vi "GetInstrumentPaths.vi"(8 "Instrument":string, 11 "Build?":bool=TRUE) -> (0 "Path To Raw Folder":path, 1 "Path To Test Folder":path, 2 "Path to csv Folder":path, 3 "Path To Instrument Folder":path, 4 "Path To TRF Folder":path)   [LabVIEW 2022 SP3]
uses:
  Mic/Mic_Global.vi
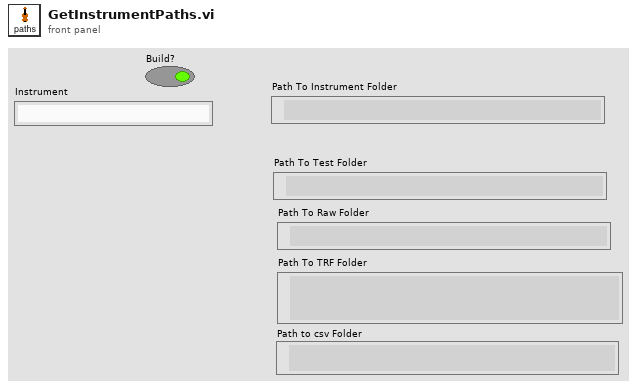
[diagram p1: front panel]
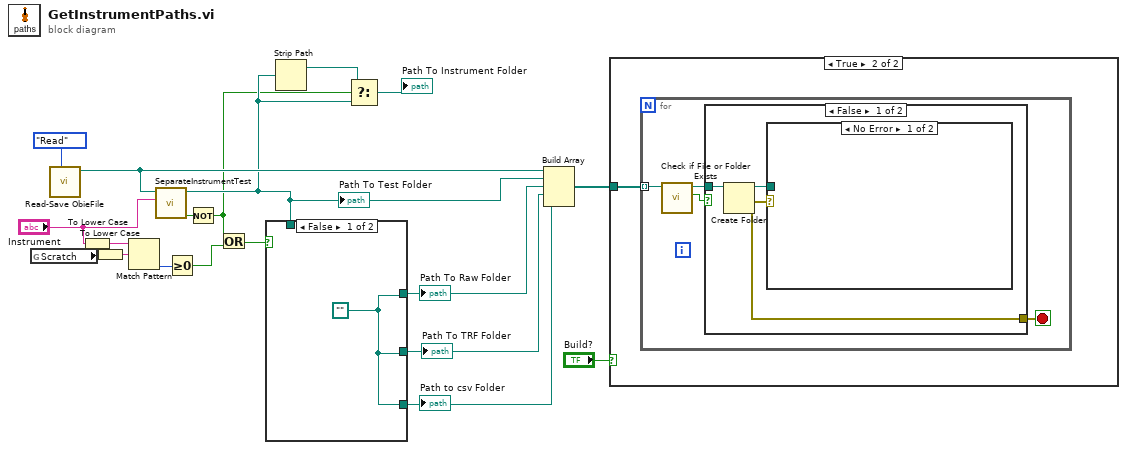
[diagram p0: block diagram]
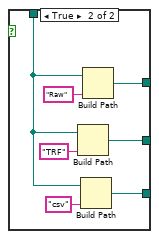
[diagram p5: hidden frame]
diagram:
  n1 = global read "Mic_Global.vi" "Scratch"() -> (w6:string)
  n2 = call "Read-Save ObieFile.vi"("Task"=enum16{"Save", "Read"}."Read") -> ("DataPath Out"=w17:path)  [unwired: 8 in, 2 out]
  n3 = To Lower Case(string="Instrument") -> (all lower case string=w2:string)
  n4 = To Lower Case(string=w6) -> (all lower case string=w1:string)
  n5 = Match Pattern(string=w2, regular expression=w1) -> (offset past match=w4:i32)  [unwired: 1 in, 3 out]
  n6 = call "SeparateInstrumentTest.vi"("Instrument"="Instrument", "path in"=w17) -> ("Single Folder?"=w11:bool, "path out"=w13:path)  [unwired: 5 in, 3 out]
  "Path To Test Folder" <- w13
  n7 = Greater Or Equal To 0?(x=w4) -> (x >= 0?=w3:bool)
  n8 = Not(x=w11) -> (.not. x?=w9:bool)
  n9 = Or(x=w9, y=w3) -> (x .or. y?=w10:bool)
  n10 = case shown="False" w10 {
    tunnel: [w20 w26] -> w16
    tunnel: [w20 w24] -> w15
    tunnel: w13 -> [_ w22]
    tunnel: [w20 w21] -> w8
    frame False {
      w20 = path ""
    }
    frame True {
      n11 = Build Path(base path=w22, name or relative path="TRF") -> (appended path=w24:path)
      n12 = Build Path(base path=w22, name or relative path="csv") -> (appended path=w21:path)
      n13 = Build Path(base path=w22, name or relative path="Raw") -> (appended path=w26:path)
    }
  }
  "Path To Raw Folder" <- w16
  "Path To TRF Folder" <- w15
  "Path to csv Folder" <- w8
  n14 = Strip Path(path=w13) -> (stripped path=w14:path)  [unwired: 1 out]
  n15 = Select(t=w14, s=w9, f=w13) -> (s? t:f=→"Path To Instrument Folder":path)
  n16 = Build Array(w17, w13, w16, w15, w8) -> (w19:path[])
  n17 = case shown="True" "Build?" {
    tunnel: w19 -> [_ w28]
    frame False {
    }
    frame True {
      n18 = for {
        tunnel: w28 -> [w30] mode=indexing
        stop <- w29 stop-if-true
        n19 = call <vilib>:"Check if File or Folder Exists.vi"("path"=w30) -> ("file or folder exists?"=w31:bool, "dup path"=w32:path)  [unwired: 8 in, 1 out]
        n20 = case shown="False" w31 {
          tunnel: w32 -> [w35 _]
          tunnel: [w33 _] -> w29
          frame False {
            n21 = Create Folder(path (use dialog)=w35) -> (created path=w34:path, error out=w33:errorcluster)  [unwired: 2 in, 1 out]
            n22 = case shown="No Error" w33 {
              tunnel: w34 -> [_ _]
              frame No Error {
              }
              frame Error {
              }
            }
          }
          frame True {
          }
        }
      }
    }
  }
